vi "Turret_Set.vi"   [LabVIEW 2019]
uses:
  Turret_States.ctl
  Globals/Turret_Globals.vi
types:
  T1 = typedef "Turret_States.ctl" = enum16{"Manual_Percent_Voltage", "Manual_Speed_Control", "Auto-Target"}
  T2 = typedef "Turret_Cluster.ctl" = cluster{"Auto-Target?":bool, "Control_State":T1, "Turret_Spin_Speed":dbl, "Turret_Spin_Speed_Control?":bool}
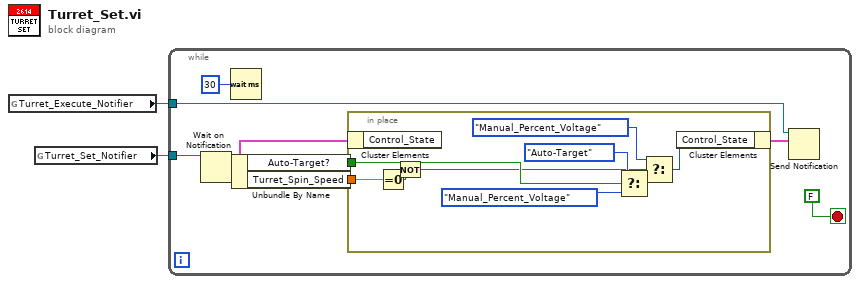
[diagram p0: block diagram]
diagram:
  n1 = global read "Turret_Globals.vi" "Turret_Execute_Notifier"() -> (w1:refnum<notifier>)
  n2 = global read "Turret_Globals.vi" "Turret_Set_Notifier"() -> (w2:refnum<notifier>)
  n3 = while {
    tunnel: w2 -> [w8]
    tunnel: w1 -> [w6]
    stop <- FALSE stop-if-true
    n4 = Wait on Notification(notifier=w8) -> (notification=w5:T2)  [unwired: 3 in, 3 out]
    n5 = Wait (ms)(milliseconds to wait=u32 30) -> ()  [unwired: 1 out]
    n6 = Unbundle By Name(w5) -> ("Auto-Target?"=w4:bool, "Turret_Spin_Speed"=w3:dbl)
    n7 = in-place {
      in-place-border: w4 -> [w17]
      in-place-border: w3 -> [w14]
      n8 = in-place-cluster #1(w5) -> ()  [unwired: 1 out]
      n9 = Equal To 0?(x=w14) -> (x = 0?=w13:bool)
      n10 = Not(x=w13) -> (.not. x?=w12:bool)
      n11 = Select(t=Turret_States."Auto-Target" ("Control_State"), s=w17, f=Turret_States."Manual_Percent_Voltage" ("Control_State")) -> (s? t:f=w16:T1)
      n12 = Select(t=Turret_States."Manual_Percent_Voltage", s=w12, f=w16) -> (s? t:f=w11:T1)
      n13 = in-place-cluster #1("Control_State"=w11) -> (w7:T2)
    }
    n14 = Send Notification(notification=w7, notifier=w6) -> ()  [unwired: 1 in, 2 out]
  }
